vi "RSZVB Set IMOD Tone Distance.vi"(8 "error in (no error)":errorcluster {"code" format="%.0x"}, 9 "Tone Distance (1.0e6 Hz)":dbl=1000000.0 format="%^.3e", 10 "Channel (1)":i32=1, 11 "VISA session":refnum<visa-resource-name>) -> (0 "error out":errorcluster {"code" format="%.0x"}, 3 "dup VISA session":refnum<visa-resource-name>)   [LabVIEW 2011]
doc: "This VI defines the tone distance (frequency offset) between the upper and the lower tone.\n\nNote(s):\n\n(1) This VI is not available for R&S ZVB instrument.\n\nRemote-control command(s):\n[SENSe<Ch>:]FREQuency:IMODulation:TDIStance"
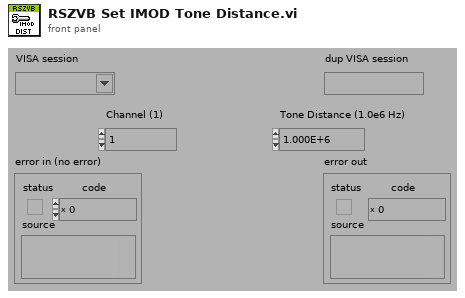
[diagram p1: front panel]
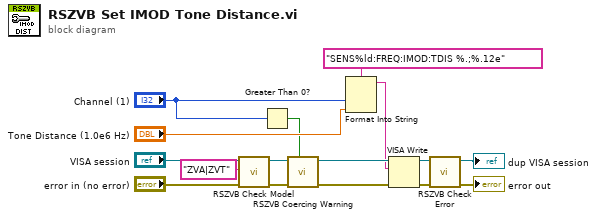
[diagram p0: block diagram]
diagram:
  n1 = call "RSZVB Check Model.vi"("error in (no error)"="error in (no error)", "Model"="ZVA|ZVT", "VISA session"="VISA session") -> ("error out"=w4:errorcluster, "dup VISA session"=w5:refnum<visa-resource-name>)  [unwired: 7 in]
  n2 = Greater Than 0?(x="Channel (1)") -> (x > 0?=w13:bool)
  n3 = call "RSZVB Coercing Warning.vi"("In Range?"=w13, "error in (no error)"=w4, "VISA session"=w5) -> ("error out"=w11:errorcluster, "dup VISA session"=w12:refnum<visa-resource-name>)  [unwired: 7 in]
  n4 = Format Into String(format string="SENS%ld:FREQ:IMOD:TDIS %.;%.12e", "Channel (1)", "Tone Distance (1.0e6 Hz)") -> (resulting string=w10:string)  [unwired: 2 in, 1 out]
  n5 = VISA Write(VISA resource name=w12, write buffer=w10, error in (no error)=w11) -> (VISA resource name out=w9:refnum<visa-resource-name>, error out=w8:errorcluster)  [unwired: 1 out]
  n6 = call "RSZVB Check Error.vi"("error in (no error)"=w8, "VISA session"=w9) -> ("error out"=→"error out":errorcluster, "dup VISA session"=→"dup VISA session":refnum<visa-resource-name>)  [unwired: 8 in]
